vi "Equals.vi"(11 "Data In":i32) -> (3 "Data Out":i32)   [LabVIEW 2018]
uses:
  Core/Assert API Components/Failure Actions.ctl
  fe743f6b-a166-4854-a674-ca9283c7de7f.vi
  Core/Assert API Components/Assert API Components.lvlib
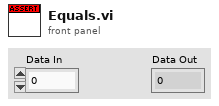
[diagram p1: front panel]
types:
  T1 = typedef "Assert API Components.lvlib/Failure Actions.ctl" = enum16{"Display Only", "Log To File", "Pause Execution", "Abort Execution"}
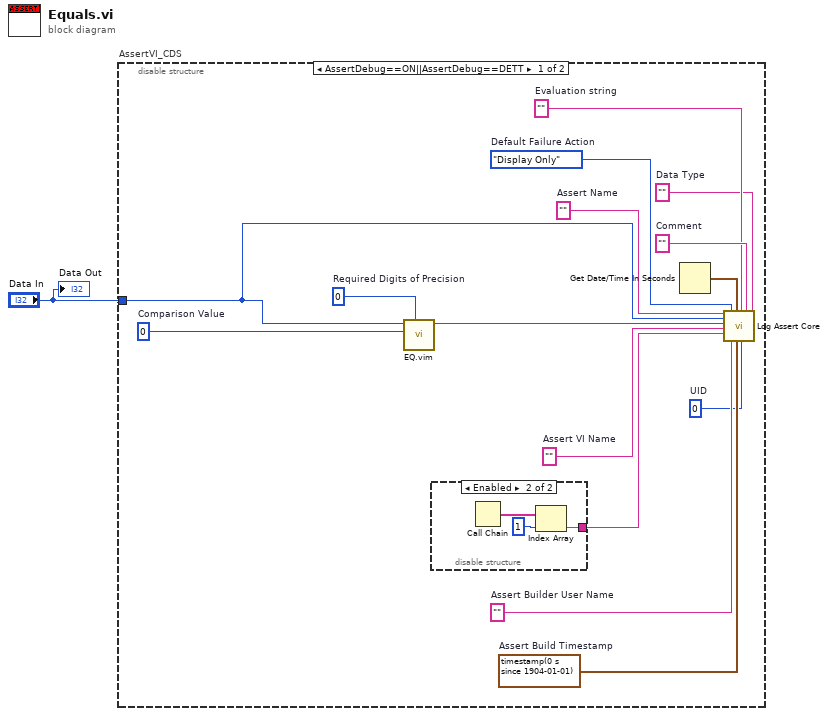
[diagram p0: block diagram]
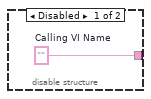
[diagram p2: hidden frame]
diagram:
  n1 = disable-structure "AssertVI_CDS" shown="AssertDebug==ON||AssertDebug==DETT" {
    disable-tunnel: "Data In" -> [w12 _]
    frame condition #0 (active) {
      w2 = 0  # Required Digits of Precision
      w4 = 0  # UID
      w6 = ""  # Assert VI Name
      w7 = timestamp(0 s since 1904-01-01)  # Assert Build Timestamp
      w8 = ""  # Assert Builder User Name
      w9 = ""  # Data Type
      w13 = ""  # Comment
      w10 = ""  # Evaluation string
      w15 = Failure_Actions."Display Only"  # Default Failure Action
      w16 = ""  # Assert Name
      w14 = 0  # Comparison Value
      n2 = call "EQ.vim"("Required Digits of Precision"=w2, "y"=w14, "x"=w12) -> ("Equal?"=w11:bool)  [unwired: 8 in]
      n3 = disable-structure shown="Enabled" {
        disable-tunnel: [w17 w18] -> w3
        frame Disabled {
          w17 = ""  # Calling VI Name
        }
        frame Enabled {
          n4 = Call Chain() -> (call chain=w19:string[])
          n5 = Index Array(array=w19, index=1) -> (element=w18:string)
        }
      }
      n6 = Get Date/Time In Seconds() -> (seconds since 1Jan1904=w5:timestamp)
      n7 = call "Log Assert Core.vi"("Assert Name"=w16, "Data Value"=w12, "Status"=w11, "Assert VI Name"=w6, "Calling VI Name"=w3, "Failure Action"=w15, "Assert Builder User Name"=w8, "Last Update"=w5, "Assert Build Timestamp"=w7, "Evaluation String"=w10, "Assert VI UID"=w4, "Comment"=w13, "Data Type"=w9) -> ()  [unwired: 7 in]
    }
    frame condition #1 {
    }
  }
  "Data Out" <- "Data In"
